vi "Destroy RPC Engine Loop Stop Notifier.vi"(8 "error in (no error)":errorcluster) -> (0 "error out":errorcluster)   [LabVIEW 2020, in "JSON-RPC Lib.lvlib" / "JSONRPC Server.lvclass"]
uses:
  JSONRPC Server.lvclass
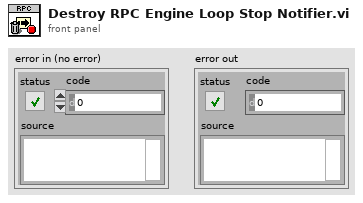
[diagram p1: front panel]
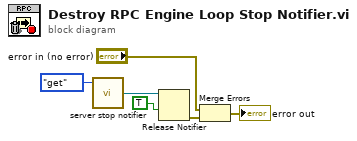
[diagram p0: block diagram]
diagram:
  n1 = call "server stop notifier.vi"("action"=enum16{"get", "set"}."get") -> ("notifier out"=w5:refnum<notifier>)  [unwired: 2 in]
  n2 = Release Notifier(notifier=w5, force destroy? (F)=TRUE ("notification")) -> (error out=w3:errorcluster)  [unwired: 1 in, 2 out]
  n3 = Merge Errors("error in (no error)", w3) -> (→"error out":errorcluster)
